vi "PCI1220U停止.vi"(11 "AxisHandle IN":u32) -> (2 "完成":bool, 3 "AxisHandle OUT":u32)   [LabVIEW 2013]
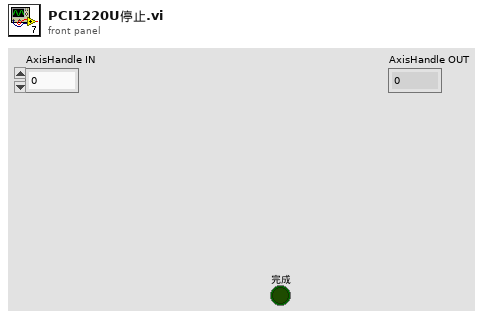
[diagram p1: front panel]
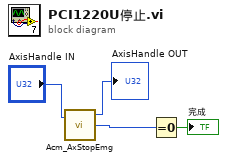
[diagram p0: block diagram]
diagram:
  n1 = call <userlib>:"Acm_AxStopEmg.vi"("AxisHandle"="AxisHandle IN") -> ("ReturnValue"=w1:u32, "AxisHandle"=→"AxisHandle OUT":u32)  [unwired: 1 in, 1 out]
  n2 = Equal To 0?(x=w1) -> (x = 0?=→"完成":bool)
